vi "Start Module.vi"(6 "Show Main VI Diagram on Init (F)":bool, 7 "Panel":refnum<class "Panel.lvclass"> caption="Panel (Window)", 8 "error in (no error)":errorcluster) -> (0 "error out":errorcluster, 1 "Wait for Event Sync?":bool, 2 "N4L_PSM3750_Interface Broadcast Events":T1, 3 "Module Was Already Running?":bool, 4 "Module Name":string)   [LabVIEW 2025, in "N4L_PSM3750_Interface.lvlib"]
doc: "Launches the Module Main.vi.\n_____\nBased on Delacor QMH Project Template 3.1.0.34.\n\n<b>Note:</b> This VI was modified by the <b>Validate DQMH Module</b> tool to add the 'Show Main VI Diagram on Init' functionality included in DQMH 6.1.\n\nThe <b>Validate DQMH Module</b> tool added a 'Module Name' output to this VI."
uses:
  N4L_PSM3750_Interface.lvlib
  Broadcast Events--cluster.ctl
  Did Init Argument--cluster.ctl
  Status Updated Argument--cluster.ctl
  Error Reported Argument--cluster.ctl
  Stop Argument--cluster.ctl
  Get Module Execution Status Argument--cluster.ctl
  Broadcast State Argument--cluster.ctl
  <vilib>/MGI/Panel Manager/Panel/Panel/Panel.lvclass
  <vilib>/Delacor/Delacor QMH/Libraries/Module Admin_class/Delacor_lib_QMH_Module Admin.lvclass
  <vilib>/Delacor/Delacor QMH/Libraries/Module Admin_class/Delacor_lib_QMH_Module Admin.lvclass/Delacor_lib_QMH_Module Admin.ctl
  <vilib>/Delacor/Delacor QMH/Libraries/Module Admin_class/Delacor_lib_QMH_Set External Launch.vi
  <vilib>/MGI/Panel Manager/Panel/Panel/Window/Window.lvclass
  <vilib>/MGI/Panel Manager/Panel/Panel/Window/Window.vi
  <vilib>/Utility/error.llb/Error Cluster From Error Code.vi
  <vilib>/ErrorRing/Error Ring.xnode
  <vilib>/MGI/Panel Manager/Panel/Panel.lvlib
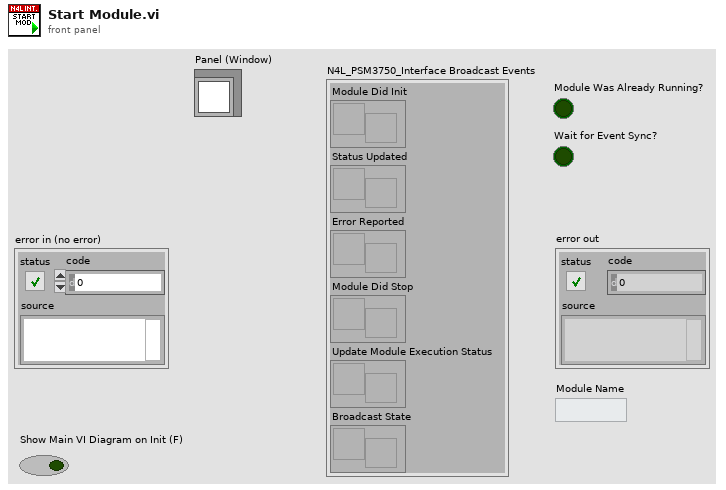
[diagram p1: front panel]
types:
  T1 = typedef "N4L_PSM3750_Interface.lvlib/Broadcast Events--cluster.ctl" = cluster{"Module Did Init":refnum<user-event>, "Status Updated":refnum<user-event>, "Error Reported":refnum<user-event>, "Module Did Stop":refnum<user-event>, "Update Module Execution Status":refnum<user-event>, "Broadcast State":refnum<user-event>}
  T2 = enum32{"Bad", "Idle", "Run top level", "Running"}
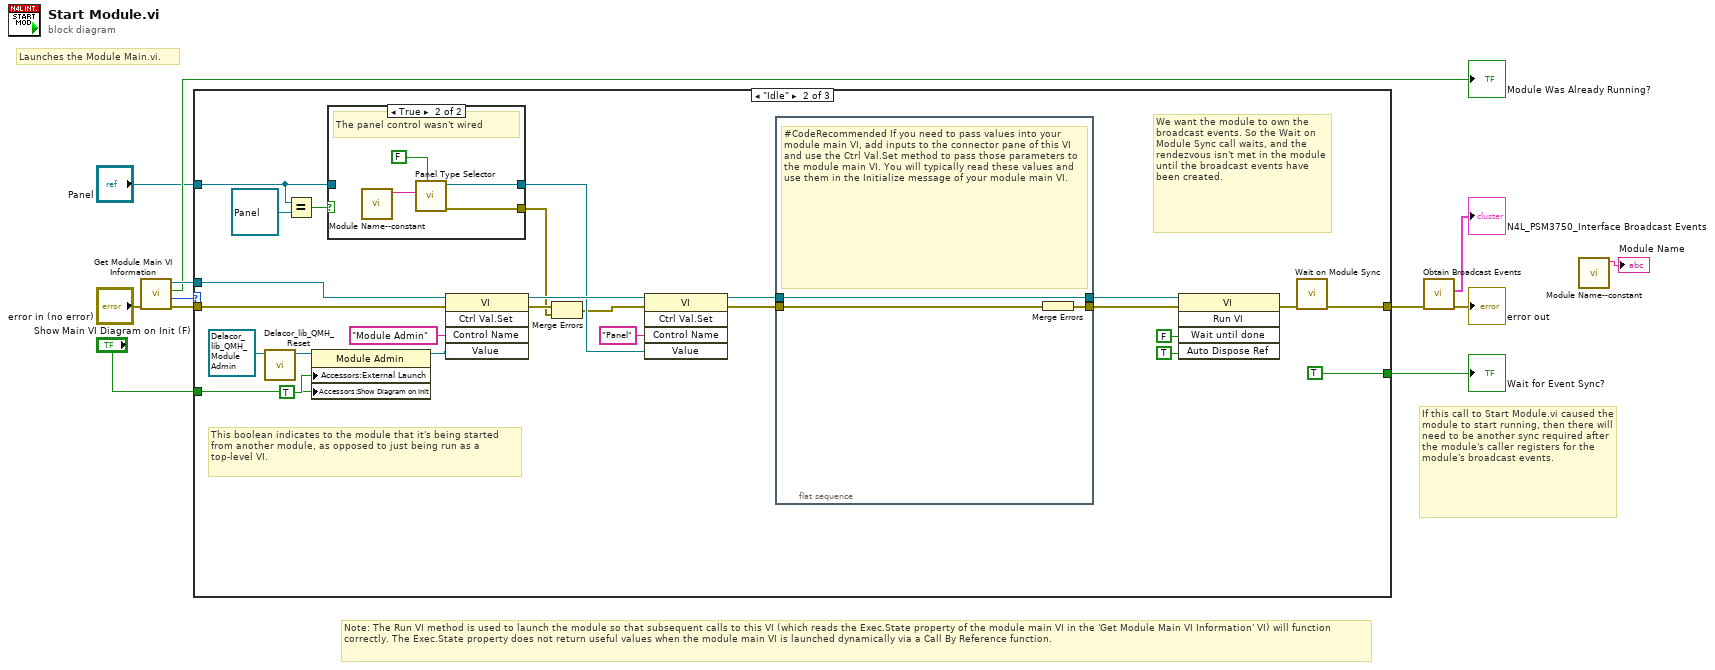
[diagram p0: block diagram]
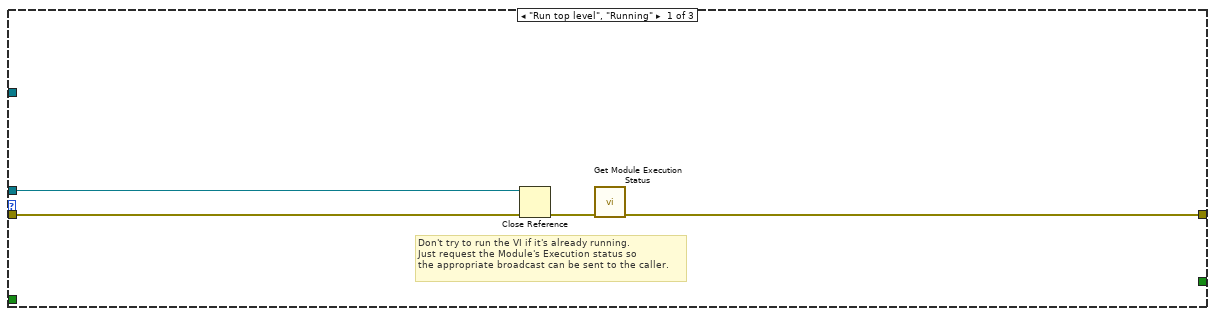
[diagram p2: hidden frame]
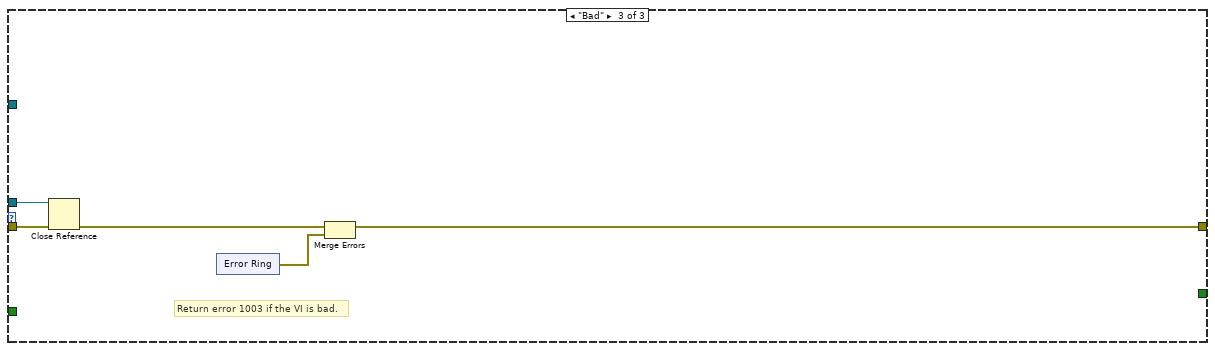
[diagram p4: hidden frame]
diagram:
  # "Note: The Run VI method is used to launch the module so that subsequent calls to this VI (which reads the Exec.State property of the module main VI in the 'Get Module Main VI Information' VI) will function correctly. The Exec.State property does not return useful values when the module main VI is launched dynamically via a Call By Reference function."
  # "If this call to Start Module.vi caused the module to start running, then there will need to be another sync required after the module's caller registers for the module's broadcast events."
  # "Launches the Module Main.vi."
  n1 = call "Get Module Main VI Information.vi"("error in (no error)"="error in (no error)") -> ("error out"=w11:errorcluster, "Execution State"=w6:T2, "Is Module Running?"=→"Module Was Already Running?":bool, "Module Main VI"=w10:refnum<vi>)  [unwired: 7 in]
  n2 = case shown="\"Idle\"" w6 {
    tunnel: w11 -> [w16 w40 w55]
    tunnel: w10 -> [w15 w41 w54]
    tunnel: [w13 w24 w52] -> w9
    tunnel: [_ TRUE _] -> w7
    tunnel: "Panel" -> [_ w21 _]
    tunnel: "Show Main VI Diagram on Init (F)" -> [_ w17 _]
    frame "Run top level", "Running" {
      # "Don't try to run the VI if it's already running.\nJust request the Module's Execution status so\nthe appropriate broadcast can be sent to the caller."
      n3 = Close Reference(reference=w15, error in (no error)=w16) -> (error out=w14:errorcluster)
      n4 = call "Get Module Execution Status.vi"("error in (no error)"=w14) -> ("error out"=w13:errorcluster)  [unwired: 10 in]
    }
    frame "Idle" {
      # "We want the module to own the broadcast events. So the Wait on Module Sync call waits, and the rendezvous isn't met in the module until the broadcast events have been created."
      # "This boolean indicates to the module that it's being started from another module, as opposed to just being run as a top-level VI."
      n5 = call-dynamic "Delacor_lib_QMH_Reset.vi"("Mod Admin in"=refnum<class "Delacor_lib_QMH_Module Admin.lvclass"> refnum) -> ("Mod Admin out"=w36:refnum<class "Delacor_lib_QMH_Module Admin.lvclass">)  [unwired: 9 in, 1 out]
      n6 = Equal?(x=w21, y=refnum<class "Panel.lvclass"> refnum) -> (x = y?=w22:bool)
      n7 = property class="Module Admin"(reference=w36, "Accessors:External Launch"=TRUE, "Accessors:Show Diagram on Init"=w17) -> (reference out=w33:refnum<class "Delacor_lib_QMH_Module Admin.lvclass">)  [unwired: 1 in, 1 out]
      n8 = case shown="True" w22 {
        tunnel: w21 -> [w43 _]
        tunnel: [w43 w47] -> w20
        tunnel: [_ w44] -> w18
        frame False {
          # "A panel object was wired in."
        }
        frame True {
          # "The panel control wasn't wired"
          n9 = call "Module Name--constant.vi"() -> ("Module Name"=w45:string)  [unwired: 11 in]
          n10 = call-poly <vilib>:"Panel Type Selector.vi"("Autoshow? (T)"=FALSE, "Default Title"=w45) -> ("error out"=w44:errorcluster, "Window out"=w47:refnum<class "Window.lvclass">)  [unwired: 8 in]
        }
      }
      n11 = invoke class="VI" method="Ctrl Val.Set"(reference=w41, error in=w40, "Control Name"="Module Admin", "Value"=w33) -> (reference out=w29:refnum<vi>, error out=w28:errorcluster)  [unwired: 1 in, 3 out]
      n12 = Merge Errors(w28, w18) -> (w19:errorcluster)
      n13 = invoke class="VI" method="Ctrl Val.Set"(reference=w29, error in=w19, "Control Name"="Panel", "Value"=w20) -> (reference out=w27:refnum<vi>, error out=w26:errorcluster)  [unwired: 1 in, 3 out]
      n14 = flat-sequence {
        tunnel: w27 -> [w50]
        tunnel: [w50] -> w32
        tunnel: w26 -> [w49]
        tunnel: [w48] -> w31
        frame #0 {
          # "#CodeRecommended If you need to pass values into your module main VI, add inputs to the connector pane of this VI and use the Ctrl Val.Set method to pass those parameters to the module main VI. You will typically read these values and use them in the Initialize message of your module main VI."
          n15 = Merge Errors(w49) -> (w48:errorcluster)
        }
      }
      n16 = invoke class="VI" method="Run VI"(reference=w32, error in=w31, "Wait until done"=FALSE ("Wait Until Done"), "Auto Dispose Ref"=TRUE ("Auto Dispose Reference")) -> (error out=w25:errorcluster)  [unwired: 1 in, 4 out]
      n17 = call "Wait on Module Sync.vi"("error in (no error)"=w25) -> ("error out"=w24:errorcluster)  [unwired: 10 in]
    }
    frame "Bad" {
      # "Return error 1003 if the VI is bad."
      n18 = Close Reference(reference=w54, error in (no error)=w55) -> (error out=w53:errorcluster)
      n19 = xnode "Error Ring"() -> ("error out"=w51:errorcluster)
      n20 = Merge Errors(w53, w51) -> (w52:errorcluster)
    }
  }
  "Wait for Event Sync?" <- w7
  n21 = call "Obtain Broadcast Events.vi"("error in (no error)"=w9) -> ("error out"=→"error out":errorcluster, "N4L_PSM3750_Interface Broadcast Events"=→"N4L_PSM3750_Interface Broadcast Events":T1)  [unwired: 9 in]
  n22 = call "Module Name--constant.vi"() -> ("Module Name"=→"Module Name":string)  [unwired: 11 in]
